vi "Frame Data.vi"() -> ()   [LabVIEW 2016]
panel:
  in  "Most Recent Frame":u8[](array[numeric])
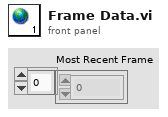
[diagram p1: front panel]
diagram:
